vi "Demo.vi"() -> ()   [LabVIEW 2014, in "K_S30c_dll.lvlib"]
uses:
  K_S30c_dll.lvlib
panel:
  out "数组":dbl[](array[numeric])
  out "Actual address 2":u8
  in  "get act addr":bool
  in  "Read out n devices":bool
  in  "Stopp":bool
  out "error out":errorcluster
  in  "Online":bool caption="Read cont.\nvalue"
  in  "Channel":enum16{"CH0", "P1", "P2", "T", "TOB1", "TOB2"}(ring)=enum."P1"
  # "using comm addr 250:\nconnect only one Transmitter!"
  # "using the comm. addr"
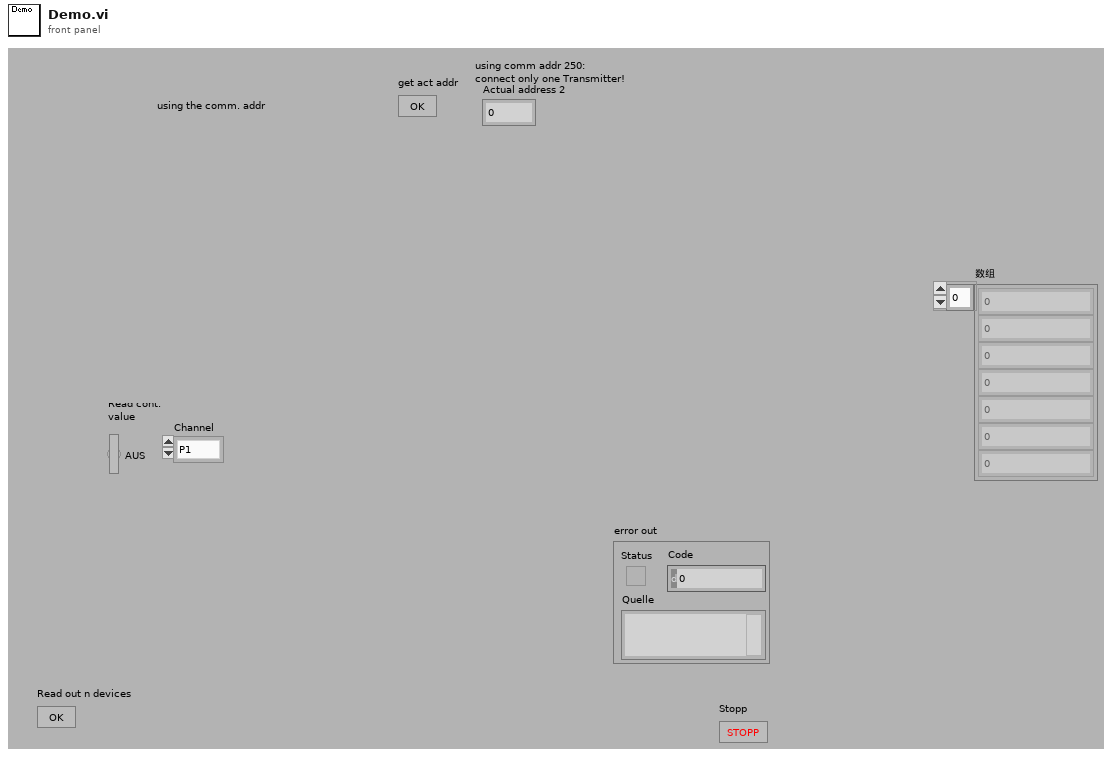
[diagram p1: front panel]
types:
  T1 = cluster{"COM":i16, "Baudrate":enum16{"9600", "115200"}, "Echo":bool, "Timeout":u32}
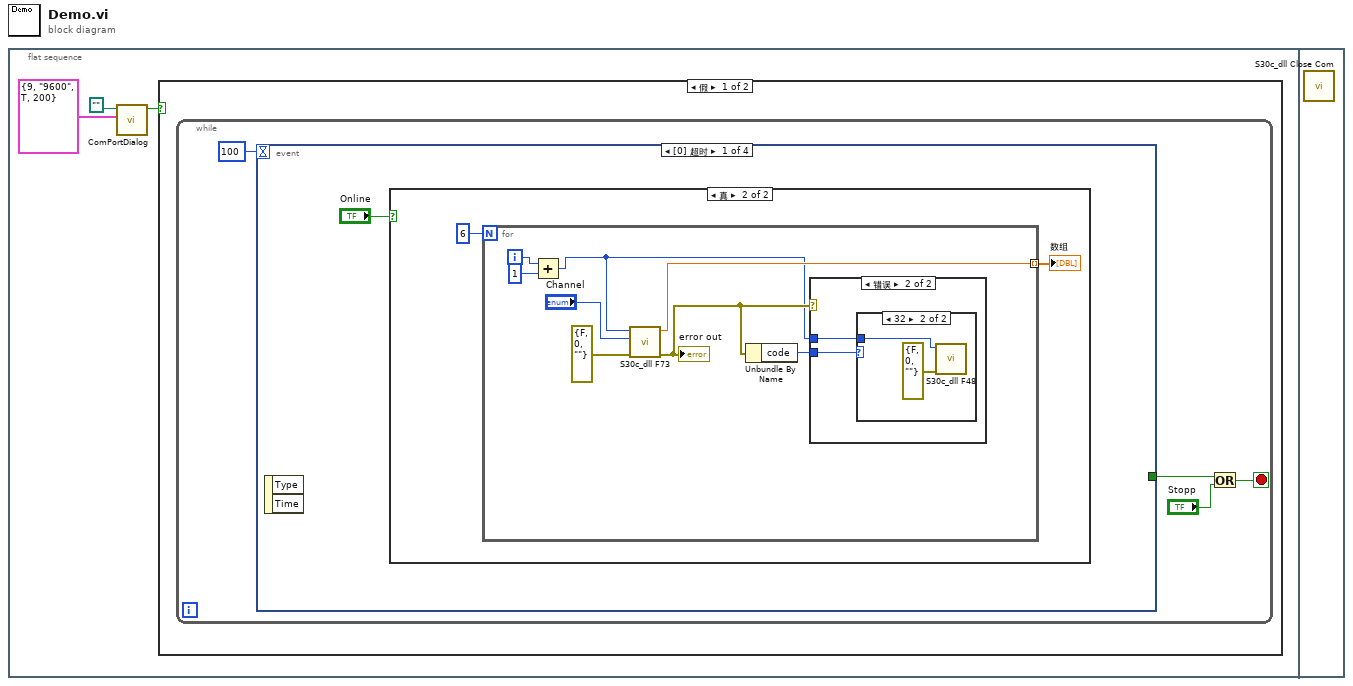
[diagram p0: block diagram]
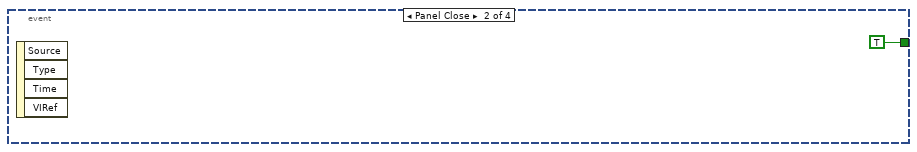
[diagram p5: hidden frame]
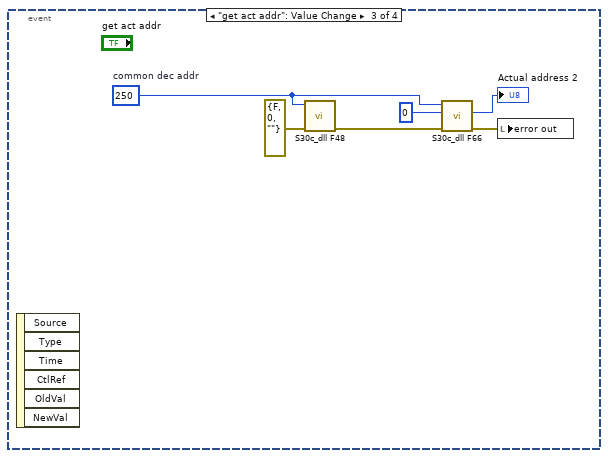
[diagram p6: hidden frame]
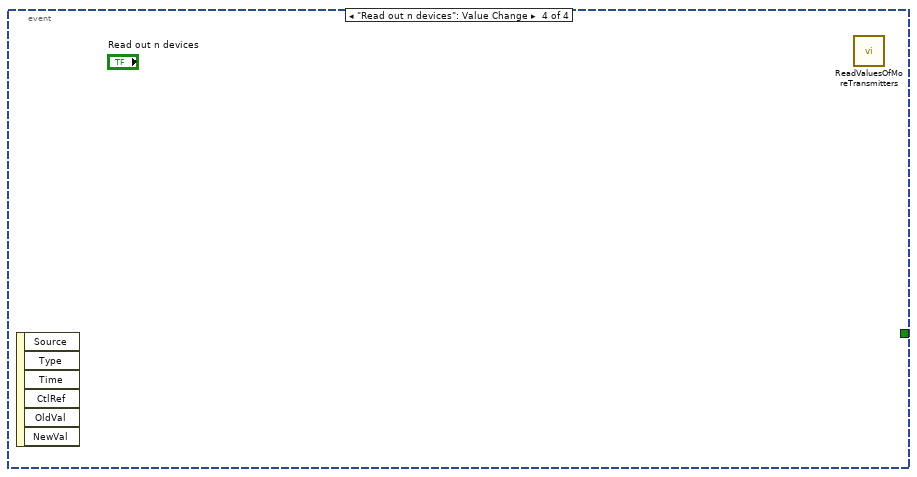
[diagram p7: hidden frame]
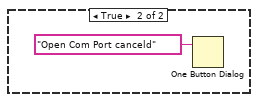
[diagram p8: hidden frame]
diagram:
  n1 = flat-sequence {
    frame #0 {
      n2 = call "ComPortDialog.vi"("Com-Einst. in"=T1 {"COM"=9, "Baudrate"=enum."9600", "Echo"=TRUE, "Timeout"=200}, "ini-File"=path "") -> ("Abbruch"=w2:bool)  [unwired: 7 in, 2 out]
      n3 = case shown="假" w2 {
        frame False {
          n4 = while {
            stop <- w4 stop-if-true
            n5 = event shown="[0] 超时" {
              selector: _ -> [_ _ _ _]
              dyn-events: _ -> [_ _ _ _]
              timeout: 100 -> [_ _ _ _]
              tunnel: [_ TRUE _ _] -> w5
              event Timeout {
                n6 = event-data() -> ()  [unwired: 1 in, 2 out]
                n7 = case shown="真" "Online" {
                  frame False {
                  }
                  frame True {
                    n8 = for {
                      N: 6 -> [_]
                      tunnel: [w14] -> w9 mode=indexing
                      i -> [w13]
                      n9 = Add(x=w13, y=1) -> (x+y=w11:i32)
                      n10 = call "S30c_dll F73.vi"("error in"=errorcluster {"status"=FALSE, "code"=0, "source"=""}, "Channel"="Channel", "Dev Addr"=w11) -> ("error out"=w18:errorcluster, "Value"=w14:sgl)  [unwired: 2 in, 1 out]
                      "error out" <- w18
                      n11 = Unbundle By Name(w18) -> ("code"=w17:i32)
                      n12 = case shown="错误" w18 {
                        tunnel: w17 -> [_ w20]
                        tunnel: w11 -> [_ w19]
                        frame No Error {
                        }
                        frame Error {
                          n13 = case shown="32" w20 {
                            tunnel: w19 -> [_ w21]
                            frame 0, Default {
                            }
                            frame 32 {
                              n14 = call "S30c_dll F48.vi"("error in"=errorcluster {"status"=FALSE, "code"=0, "source"=""}, "Dev Addr"=w21) -> ()  [unwired: 3 in, 3 out]
                            }
                          }
                        }
                      }
                    }
                    "数组" <- w9
                  }
                }
              }
              event Panel Close {
                n15 = event-data() -> ()  [unwired: 1 in, 4 out]
              }
              event "get act addr": Value Change {
                w24 = u8 250  # common dec addr
                n16 = event-data() -> ()  [unwired: 1 in, 6 out]
                n17 = call "S30c_dll F48.vi"("error in"=errorcluster {"status"=FALSE, "code"=0, "source"=""}, "Dev Addr"=w24) -> ("error out"=w26:errorcluster)  [unwired: 3 in, 2 out]
                n18 = call "S30c_dll F66.vi"("error in"=w26, "New address"=u8 0, "Dev Addr"=w24) -> ("error out"=w27:errorcluster, "Actual address"=→"Actual address 2":u8)  [unwired: 3 in]
                n19 = local write "error out"(w27) -> ()
              }
              event "Read out n devices": Value Change {
                n20 = event-data() -> ()  [unwired: 1 in, 6 out]
                n21 = call "ReadValuesOfMoreTransmitters.vi"() -> ()  [unwired: 1 in]
              }
            }
            n22 = Or(x=w5, y="Stopp") -> (x .or. y?=w4:bool)
          }
        }
        frame True {
          n23 = One Button Dialog(message="Open Com Port canceld" ("Nachricht")) -> ()  [unwired: 1 in, 1 out]
        }
      }
    }
    frame #1 {
      n24 = call "S30c_dll Close Com.vi"() -> ()  [unwired: 7 in, 1 out]
    }
  }
